vi "Actor Core.vi"(8 "Error In":errorcluster, 11 "BNT_XtGraph in":refnum<class "BNT_XtGraph.lvclass">) -> (0 "Error Out":errorcluster, 3 "Actor out":refnum<class "Actor.lvclass">)   [LabVIEW 2018, in "BNT_XtGraph.lvlib" / "BNT_XtGraph.lvclass"]
doc: "(<B>Filename</B>: Actor Framework.lvlib:Actor.lvclass:Actor Core.vi)\n\nReceives messages to the actor, reacts to them, and initiates any error handling that may shut the actor down.\n\nDescendant classes may override this VI to append parallel tasks for the actor to complete while it handles messages. Overrides use the Call Parent Method node."
uses:
  BNT_XtGraph.lvclass
  C:/Users/Holger/Documents/LVP/HEITRONICS/TempCtrl/Packages/CSPP_Core/Actors/CSPP_BaseActor/CSPP_BaseActor.lvclass
  C:/Program Files (x86)/National Instruments/LabVIEW 2018/vi.lib/ActorFramework/Actor/Actor.lvclass
  <vilib>/ActorFramework/Actor/Actor.lvclass
  BNT_XtGraph.lvclass/BNT_XtGraph.ctl
  CSPP_Core/Actors/CSPP_BaseActor/CSPP_BaseActor.lvclass/CSPP_BaseActor.ctl
  <vilib>/ActorFramework/Actor/Actor.lvclass/Actor.ctl
  <vilib>/ActorFramework/Message Enqueuer/Message Enqueuer.lvclass/Message Enqueuer.ctl
  CSPP_Core/Messages/CSPP_AsyncCallbackMsg/CSPP_AsyncCallback Msg.lvclass/CSPP_AsyncCallback Msg.ctl
  CSPP_Core/Actors/CSPP_BaseActor/Read Object Name.vi
  <vilib>/ActorFramework/Message Enqueuer/Init from Existing Queue.vi
  <vilib>/ActorFramework/Message Enqueuer/Enqueue.vi
  CSPP_Core/Messages/CSPP_AsyncCallbackMsg/Read Error.vi
  CSPP_Core/Messages/CSPP_AsyncCallbackMsg/Write Callback Queue.vi
  <vilib>/ActorFramework/Message Enqueuer/Equals Not A Refnum.vi
  BNT_XtGraph Messages/Clear History Msg/Clear History Msg.lvclass
  C:/Users/Holger/Documents/LVP/HEITRONICS/TempCtrl/Packages/CSPP_Core/Messages/CSPP_AsyncCallbackMsg/CSPP_AsyncCallback Msg.lvclass
  C:/Program Files (x86)/National Instruments/LabVIEW 2018/vi.lib/ActorFramework/Message/Message.lvclass
  CSPP_Core/Messages/CSPP_AsyncCallbackMsg/Read Actor Enqueuer.vi
  CSPP_Core/Libraries/Utilities/Error Cluster from Error Code.vi
  <vilib>/ActorFramework/Message Priority Queue/Priority Enqueue.vi
  <vilib>/ActorFramework/Message Enqueuer/Message Enqueuer.lvclass
  CSPP_Core/Actors/CSPP_BaseActor/CSPP_BaseActor.lvclass
  CSPP_Core/Libraries/Utilities/CSPP_Utilities.lvlib
panel:
  out "X-t Graph":T1(graph)
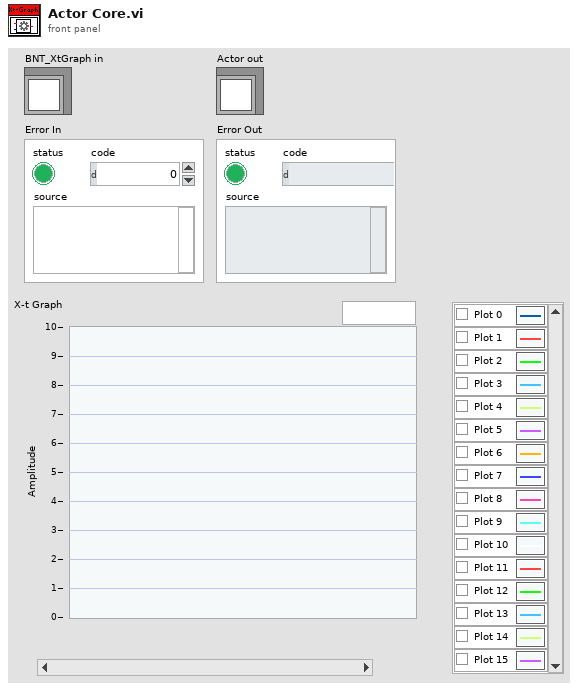
[diagram p1: front panel]
types:
  T1 = cluster{"X-t Value Pairs":cluster{"Time Stamp":timestamp, "Value":dbl}[]}[]
  T2 = enum32{"Invalid", "Standard", "Closed", "Hidden", "Minimized", "Maximized"}
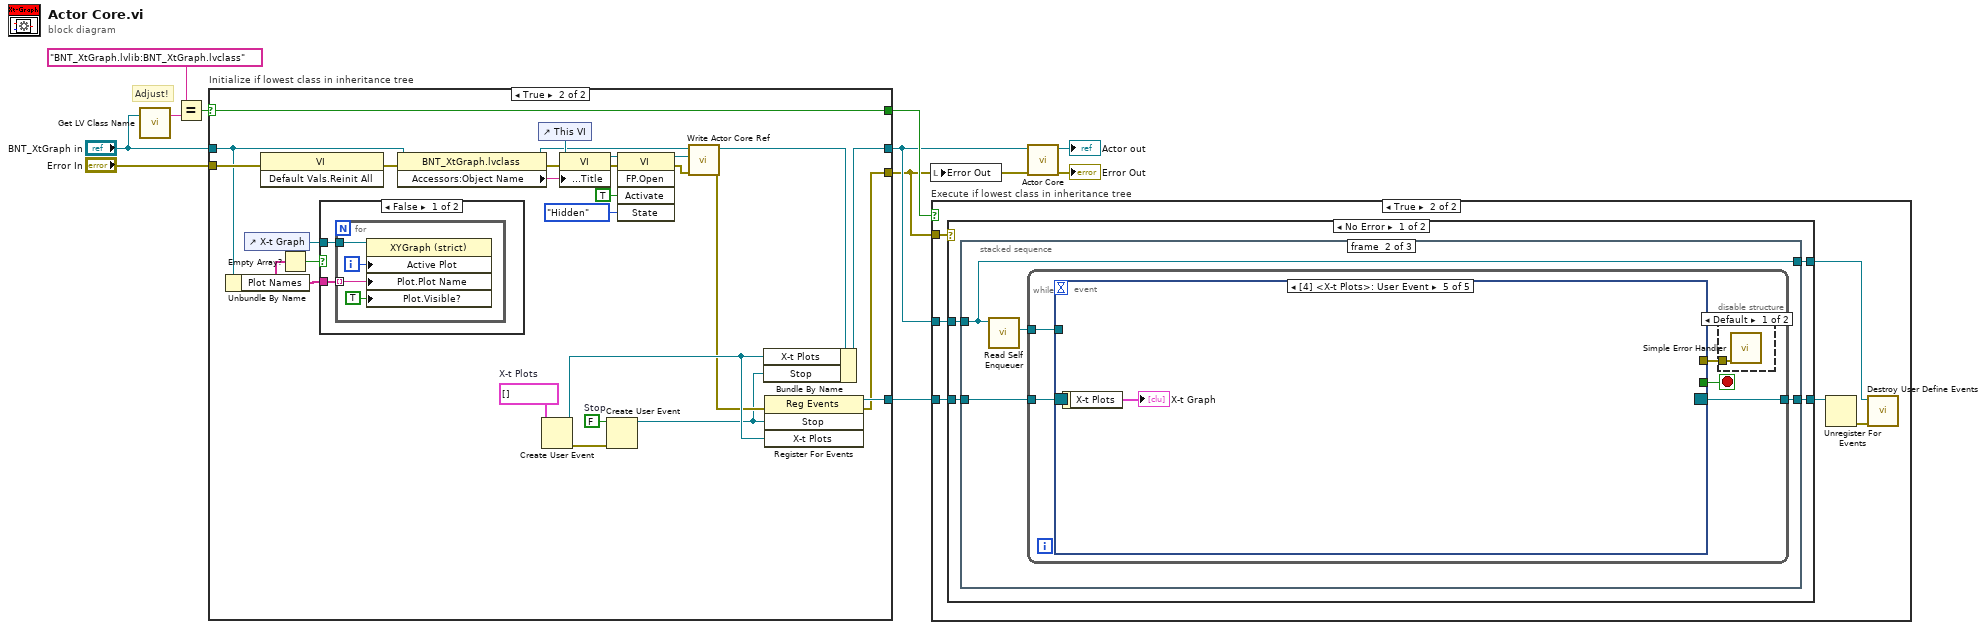
[diagram p0: block diagram]
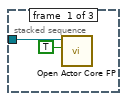
[diagram p5: hidden frame]
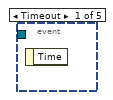
[diagram p6: hidden frame]
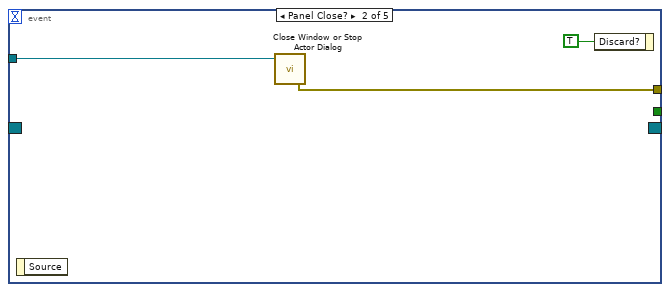
[diagram p7: hidden frame]
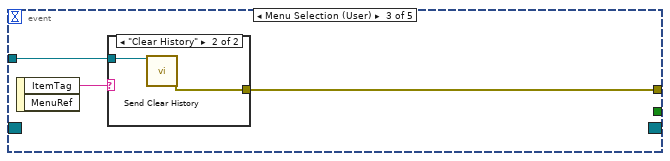
[diagram p8: hidden frame]
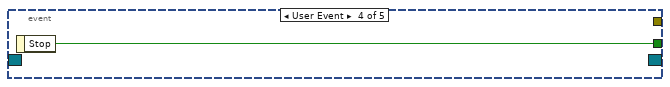
[diagram p10: hidden frame]
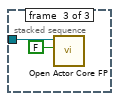
[diagram p12: hidden frame]
diagram:
  # "Adjust!"
  n1 = call <vilib>:"Get LV Class Name.vi"("object"="BNT_XtGraph in") -> ("class name"=w9:string)  [unwired: 9 in, 1 out]
  n2 = Equal?(x="BNT_XtGraph.lvlib:BNT_XtGraph.lvclass" ("class name"), y=w9) -> (x = y?=w7:bool)
  n3 = case "Initialize if lowest class in inheritance tree" shown="True" w7 {
    selector: w7 -> [w14 w39]
    tunnel: "Error In" -> [w12 w30]
    tunnel: "BNT_XtGraph in" -> [w13 w18]
    tunnel: [w13 w25] -> w4
    tunnel: [w12 w22] -> w3
    tunnel: [w14 w39] -> w6
    tunnel: [_ w27] -> w5
    frame False {
    }
    frame True {
      w20 = FALSE  # Stop
      w28 = T1 []  # X-t Plots
      n4 = Unbundle By Name(w18) -> ("Plot Names"=w15:string[])
      n5 = control-ref of="X-t Graph"() -> (w17:refnum<vi>)
      n6 = invoke class="VI" method="Default Vals.Reinit All"(error in=w30) -> (error out=w29:errorcluster)  [unwired: 2 in, 2 out]
      n7 = Empty Array?(array=w15) -> (empty?=w16:bool)
      n8 = case shown="False" w16 {
        tunnel: w17 -> [w43 _]
        tunnel: w15 -> [w42 _]
        frame False {
          n9 = for {
            tunnel: w43 -> [w47]
            tunnel: w42 -> [w46] mode=indexing
            i -> [w45]
            n10 = property class="XYGraph (strict)"(reference=w47, "Active Plot"=w45, "Plot.Plot Name"=w46, "Plot.Visible?"=TRUE ("Plot.Visible")) -> ()  [unwired: 1 in, 2 out]
          }
        }
        frame True {
        }
      }
      n11 = property class="BNT_XtGraph.lvclass"(reference=w18, error in=w29) -> (reference out=w31:refnum<class "BNT_XtGraph.lvclass">, error out=w33:errorcluster, "Accessors:Object Name"=w32:string)
      n12 = control-ref of="This VI"() -> (w36:refnum<vi>)
      n13 = Create User Event(user event datatype=w28) -> (user event=w24:refnum<user-event>, error out=w21:errorcluster)  [unwired: 1 in]
      n14 = property class="VI"(reference=w36, error in=w33, "Front Panel.Title"=w32) -> (reference out=w35:refnum<vi>, error out=w34:errorcluster)
      n15 = Create User Event(user event datatype=w20, error in=w21) -> (user event=w19:refnum<user-event>)  [unwired: 1 out]
      n16 = invoke class="VI" method="FP.Open"(reference=w35, error in=w34, "Activate"=TRUE ("Activate?"), "State"=T2."Hidden") -> (reference out=w38:refnum<vi>, error out=w37:errorcluster)  [unwired: 1 in, 3 out]
      n17 = call "Write Actor Core Ref.vi"("error in (no error)"=w37, "Actor Core Ref"=w38, "CSPP_BaseActor in"=w31) -> ("error out"=w23:errorcluster, "CSPP_BaseActor out"=w26:refnum<class "BNT_XtGraph.lvclass">)  [unwired: 7 in]
      n18 = Bundle By Name(cluster=w26, "X-t Plots"=w24, "Stop"=w19) -> (w25:refnum<class "BNT_XtGraph.lvclass">)
      n19 = register-events(error in=w23, w19, w24) -> (reference out=w27:refnum<event-registration>, error out=w22:errorcluster)  [unwired: 1 in]
    }
  }
  n20 = local write "Error Out"(w3) -> ()
  n21 = case "Execute if lowest class in inheritance tree" shown="True" w6 {
    tunnel: w4 -> [_ w53]
    tunnel: w3 -> [_ w52]
    tunnel: w5 -> [_ w51]
    frame False {
    }
    frame True {
      n22 = case shown="No Error" w52 {
        tunnel: w53 -> [w57 w83]
        tunnel: w51 -> [w56 w82]
        tunnel: [w55 w82] -> w49
        tunnel: [w54 w83] -> w48
        frame No Error {
          n23 = stacked-sequence {
            tunnel: w57 -> [w59 w60 w81]
            tunnel: w56 -> [_ w62 _]
            tunnel: [_ w61 _] -> w55
            tunnel: [_ w60 _] -> w54
            frame #0 {
              n24 = call "Open Actor Core FP.vi"("Open FP (F)"=TRUE, "CSPP_BaseActor in"=w59) -> ()  [unwired: 8 in, 2 out]
            }
            frame #1 {
              n25 = call <vilib>:"Read Self Enqueuer.vi"("Actor"=w60) -> ("Self Enqueuer"=w63:refnum<class "Message Enqueuer.lvclass">)  [unwired: 10 in]
              n26 = while {
                tunnel: w62 -> [w68]
                tunnel: [w66] -> w61
                tunnel: w63 -> [w64]
                stop <- w67 stop-if-true
                n27 = event shown="[4] <X-t Plots>: User Event" {
                  selector: w68 -> [_ _ _ _ _]
                  dyn-events: [_ _ _ _ _] -> w66
                  timeout: _ -> [_ _ _ _ _]
                  tunnel: [_ _ _ w77 _] -> w67
                  tunnel: [_ w69 w72 _ _] -> w65
                  tunnel: w64 -> [_ w70 w73 _ _]
                  event Timeout {
                    n28 = event-data() -> ()  [unwired: 1 in, 1 out]
                  }
                  event Panel Close? {
                    n29 = event-data() -> ()  [unwired: 1 in, 1 out]
                    n30 = call "Close Window or Stop Actor Dialog.vi"("Self Enqueuer"=w70) -> ("Error Out"=w69:errorcluster)  [unwired: 2 in]
                    n31 = event-data("Discard?"=TRUE) -> ()  [unwired: 1 in, 1 out]
                  }
                  event Menu Selection (User) {
                    n32 = event-data() -> ("ItemTag"=w74:string)  [unwired: 1 in, 1 out]
                    n33 = case shown="\"Clear History\"" w74 {
                      tunnel: w73 -> [_ w76]
                      tunnel: [_ w75] -> w72
                      frame "False", Default {
                      }
                      frame "Clear History" {
                        n34 = call "Send Clear History.vi"("Message Enqueuer"=w76) -> ("error out"=w75:errorcluster)  [unwired: 16 in, 2 out]
                      }
                    }
                  }
                  event User Event {
                    n35 = event-data() -> ("Stop"=w77:bool)  [unwired: 1 in]
                  }
                  event User Event {
                    n36 = event-data() -> ("X-t Plots"=→"X-t Graph":T1)  [unwired: 1 in]
                  }
                }
                n37 = disable-structure shown="Default" {
                  disable-tunnel: w65 -> [w79 _]
                  frame condition #0 (active) {
                    n38 = call <vilib>:"Simple Error Handler.vi"("error in (no error)"=w79) -> ()  [unwired: 4 in, 5 out]
                  }
                  frame condition #1 {
                  }
                }
              }
            }
            frame #2 {
              n39 = call "Open Actor Core FP.vi"("Open FP (F)"=FALSE, "CSPP_BaseActor in"=w81) -> ()  [unwired: 8 in, 2 out]
            }
          }
        }
        frame Error {
        }
      }
      n40 = Unregister For Events(event registration refnum=w49) -> (error out=w50:errorcluster)  [unwired: 1 in]
      n41 = call-dynamic "Destroy User Define Events.vi"("Error In"=w50, "BNT_XtGraph in"=w48) -> ()  [unwired: 8 in, 2 out]
    }
  }
  n42 = call-parent "Actor Core.vi"("error in"=w3, "CSPP_BaseActor in"=w4) -> ("error out"=→"Error Out":errorcluster, "Actor out"=→"Actor out":refnum<class "Actor.lvclass">)  [unwired: 8 in]
